vi "Calculate Thrust.vi"(8 "error in (no error)":errorcluster, 10 "Vessel in":refnum<class "Vessel.lvclass">, 11 "Thrust Allocation in":refnum<class "Thrust Allocation.lvclass">) -> (0 "error out":errorcluster, 2 "Vessel out":refnum<class "Vessel.lvclass">, 3 "Thrust Allocation out":refnum<class "Thrust Allocation.lvclass">)   [LabVIEW 2014, in "Thrust Allocation.lvclass"]
uses:
  Thrust Allocation.lvclass
  ROV/Vessel.lvclass
  <vilib>/Analysis/Matrix/Datatypes/RealMatrix.ctl
  <vilib>/Analysis/_algsub.llb/Real PseudoInverse Matrix.vi
  <vilib>/Analysis/baseanly.llb/A x Vector.vi
  <vilib>/Analysis/Matrix/Numeric/Multiply/Multiply - RM,R.vi
  <vilib>/Analysis/Matrix/Numeric/Conversions/Matrix To Array - RM.vi
  <vilib>/imath/engines/lvmath2/RunTimeEngine/IndexRead/NIMS M($,S).vi
  <instcachedir>/0/NIMS M($,S)_3E5749BBB62E49528D4765A77F1F6D98.lvgen/NIMS M($,S)_3E5749BBB62E49528D4765A77F1F6D98_000.vi
  <vilib>/imathl/engines/lvmath/Functions/Error Handling/Create Error.vi
  <vilib>/imath/engines/lvmath2/RunTimeEngine/BuiltInFunctions/length/NIMS_length(GV).vi
  <instcachedir>/0/NIMS_length(GV)_08A3D13377FD4E4B96F5795FBF3698FA.lvgen/NIMS_length(GV)_08A3D13377FD4E4B96F5795FBF3698FA_000.vi
  <vilib>/imath/engines/lvmath2/RunTimeEngine/RangeToken/NIMS_Range_R2 - Integer.vi
  <instcachedir>/0/NIMS_Range_R2 - Integer_2D1304BAF97744E0A293025746CBADFC.lvgen/NIMS_Range_R2 - Integer_2D1304BAF97744E0A293025746CBADFC_000.vi
  <vilib>/imath/engines/lvmath2/RunTimeEngine/CommandStatement/MC_CommandStatement_break.vi
  <vilib>/imath/engines/lvmath2/RunTimeEngine/IndexRead/NIMS V(S).vi
  <instcachedir>/0/NIMS V(S)_0488751826AF41519A22953C041130DC.lvgen/NIMS V(S)_0488751826AF41519A22953C041130DC_000.vi
  <vilib>/imath/engines/lvmath2/RunTimeEngine/VariableToken/NIMS_VariableToken_CondDefinedDefinedByReplace.vi
  <instcachedir>/0/NIMS_VariableToken_CondDefinedDefinedByReplace_D162CFFC24174562A9FEA619A91E1A56.lvgen/NIMS_VariableToken_CondDefinedDefinedByReplace_D162CFFC24174562A9FEA619A91E1A56_002.vi
  <vilib>/imath/engines/lvmath2/RunTimeEngine/IndexReplace/NIMS V(S)=S.vi
  <instcachedir>/0/NIMS V(S)=S_2D52C4EC15D8415E870AEE69FB516CCA.lvgen/NIMS V(S)=S_2D52C4EC15D8415E870AEE69FB516CCA_000.vi
  <vilib>/imath/engines/lvmath2/RunTimeEngine/ErrorHandling/NIMS_Create Error From Enums.vi
  <vilib>/imath/engines/lvmath2/RunTimeEngine/VariableToken/NIMS_VariableToken_CondDefined.vi
  <instcachedir>/0/NIMS_VariableToken_CondDefined_EE8DD211A89249938CE6537267F5C9B3.lvgen/NIMS_VariableToken_CondDefined_EE8DD211A89249938CE6537267F5C9B3_005.vi
  <vilib>/imath/engines/lvmath2/RunTimeEngine/NodeEndStatement/NIMS_NodeEndStatement_Output.vi
  <instcachedir>/0/NIMS_NodeEndStatement_Output_53EC0D466D134D7ABD903AC30B43404B.lvgen/NIMS_NodeEndStatement_Output_53EC0D466D134D7ABD903AC30B43404B_005.vi
  <vilib>/imath/engines/lvmath2/RunTimeEngine/ErrorHandling/NIMS_Finalize Error.vi
  Supervisor/Supervisor.lvclass
  Thruster/Thruster.lvclass
  <vilib>/Analysis/NI_AALPro.lvlib
  <vilib>/Analysis/NI_AALBase.lvlib
  <vilib>/Analysis/Matrix/NI_Matrix.lvlib
panel:
  in  "Numeric":dbl=1.0
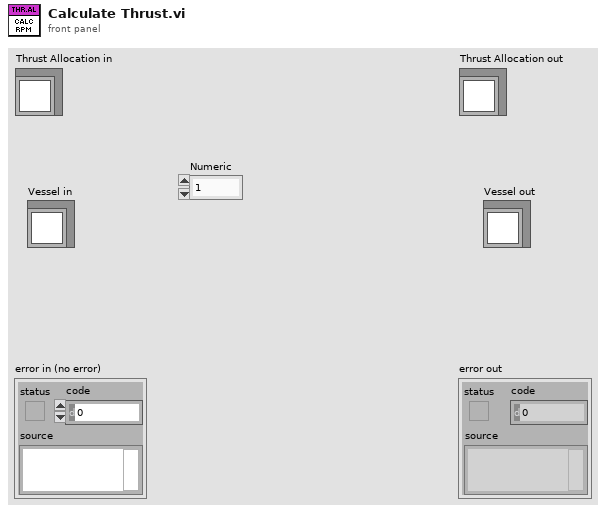
[diagram p1: front panel]
types:
  T1 = typedef "NI_Matrix.lvlib/RealMatrix.ctl" = dbl[][]
  T2 = cluster{"Measured":cluster{"Eta":dbl[], "Nu":dbl[], "Eta Dot":dbl[], "Nu Dot":dbl[]}, "Estimated":cluster{"Eta":dbl[], "Nu":dbl[], "Eta Dot":dbl[], "Nu Dot":dbl[]}, "Desired":cluster{"Eta":dbl[], "Nu":dbl[], "Eta Dot":dbl[], "Nu Dot":dbl[]}, "Previous Desired":cluster{"Eta":dbl[], "Nu":dbl[], "Eta Dot":dbl[], "Nu Dot":dbl[]}, "tau":dbl[], "Altitude":cluster{"Measured":dbl, "Estimated":dbl, "Desired":dbl, "Previous Desired":dbl, "Approximated":dbl, "grad F":dbl[]}, "rpm":dbl[], "Attitude":cluster{"Theta Measured":dbl[], "Theta Estimated":dbl[], "Omega Measured":dbl[], "Omega Estimated":dbl[], "Gyro Bias":dbl[]}}
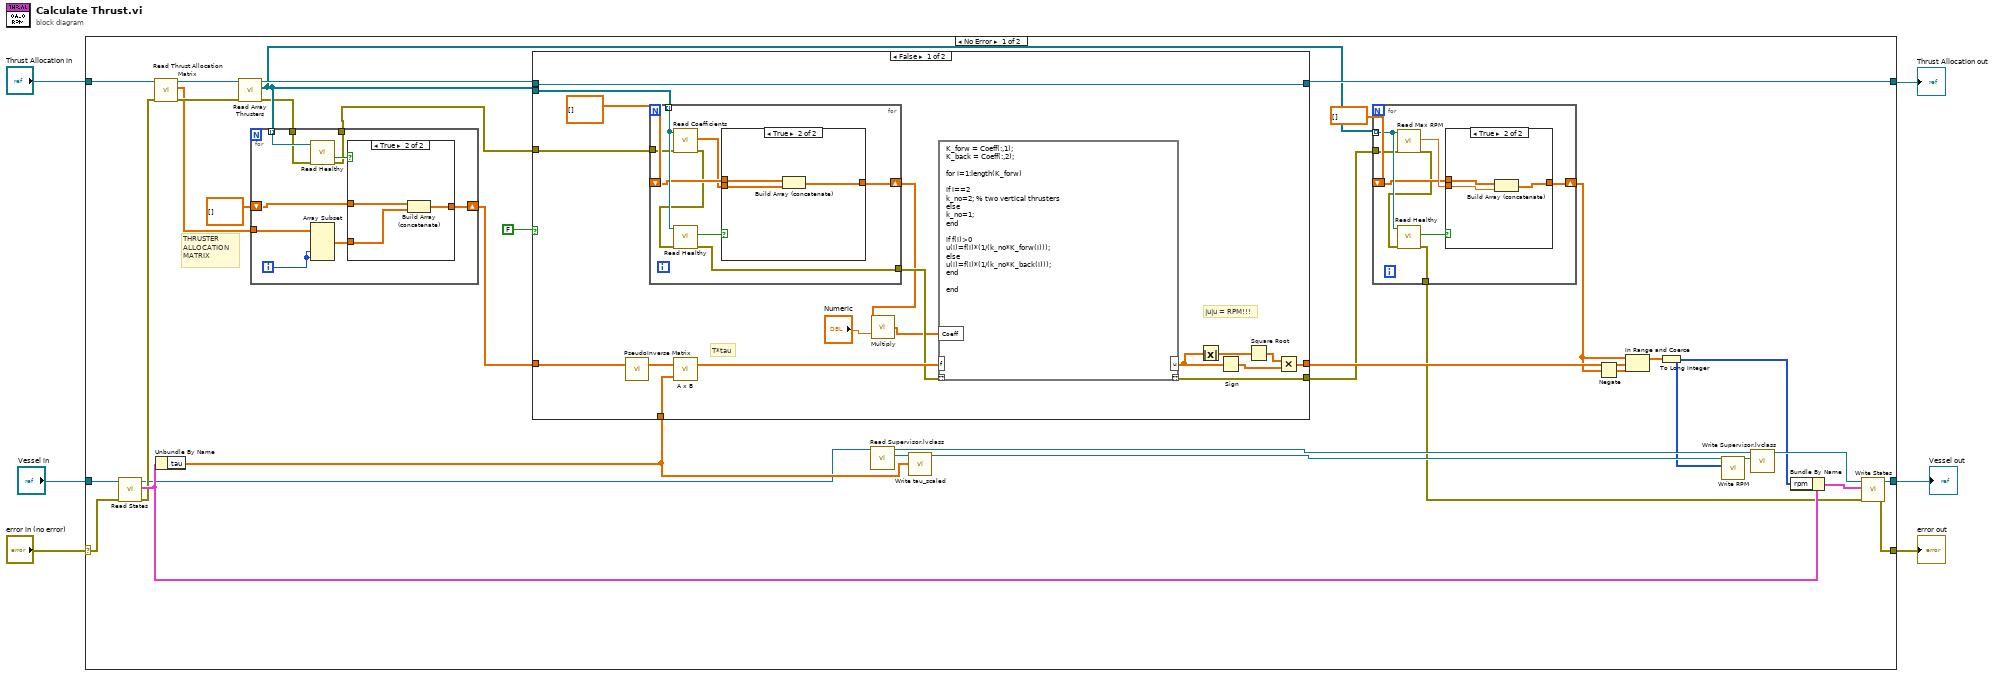
[diagram p0: block diagram]
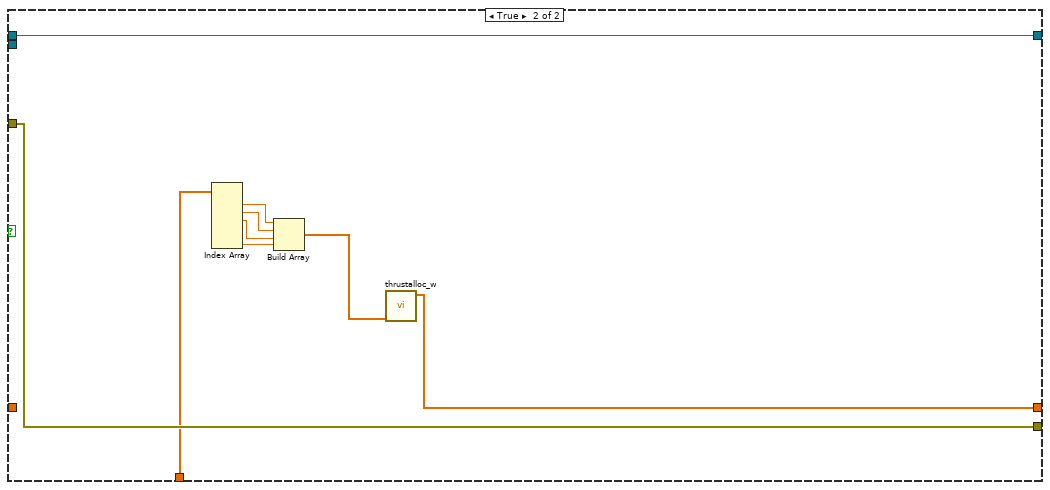
[diagram p3: hidden frame]
diagram:
  n1 = case shown="No Error" "error in (no error)" {
    selector: "error in (no error)" -> [w34 w345]
    tunnel: [w32 w345] -> w5
    tunnel: [w22 w344] -> w3
    tunnel: "Thrust Allocation in" -> [w25 w344]
    tunnel: "Vessel in" -> [w38 w343]
    tunnel: [w35 w343] -> w1
    frame No Error {
      # "THRUSTER\nALLOCATION\nMATRIX"
      n2 = call-dynamic "Read States.vi"("error in (no error)"=w34, "Vessel in"=w38) -> ("error out"=w24:errorcluster, "States"=w37:T2, "Vessel out"=w7:refnum<class "Vessel.lvclass">)  [unwired: 7 in]
      n3 = call-dynamic "Read Thrust Allocation Matrix.vi"("error in (no error)"=w24, "Thrust Allocation in"=w25) -> ("error out"=w33:errorcluster, "T"=w20:T1, "Thrust Allocation out"=w40:refnum<class "Thrust Allocation.lvclass">)  [unwired: 7 in]
      n4 = Unbundle By Name(w37) -> ("tau"=w8:dbl[])
      n5 = call "Read Array Thrusters.vi"("error in (no error)"=w33, "Thrust Allocation in"=w40) -> ("error out"=w16:errorcluster, "Array Thrusters"=w18:refnum<class "Thruster.lvclass">[], "Thrust Allocation out"=w23:refnum<class "Thrust Allocation.lvclass">)  [unwired: 7 in]
      n6 = for {
        shift-right: [w323] -> w19
        shift-left: T1 [] ("T") -> [w322]
        tunnel: w20 -> [w321]
        tunnel: w18 -> [w320] mode=indexing
        tunnel: w16 -> [w319]
        tunnel: [w318] -> w15
        i -> [w326]
        n7 = call-dynamic "Read Healthy.vi"("error in (no error)"=w319, "Thruster in"=w320) -> ("error out"=w318:errorcluster, "Healthy"=w324:bool)  [unwired: 7 in, 1 out]
        n8 = Array Subset(array=w321, index (col)=w326, length (col)=w326) -> (w325:T1)  [unwired: 2 in]
        n9 = case shown="True" w324 {
          tunnel: w325 -> [_ w330]
          tunnel: [w327 w329] -> w323
          tunnel: w322 -> [w327 w328]
          frame False {
          }
          frame True {
            n10 = Build Array (concatenate)(w328, w330) -> (w329:T1)
          }
        }
      }
      n11 = case shown="False" FALSE {
        tunnel: w8 -> [w58 w314]
        tunnel: w23 -> [w50 w317]
        tunnel: [w50 w317] -> w22
        tunnel: [w44 w315] -> w21
        tunnel: w19 -> [w55 _]
        tunnel: w18 -> [w54 _]
        tunnel: w15 -> [w53 w316]
        tunnel: [w52 w316] -> w13
        frame False {
          # "T*tau"
          # "|u|u = RPM!!!"
          n12 = call-poly <vilib>:"PseudoInverse Matrix.vi"("Input Matrix"=w55) -> ("PseudoInverse Matrix"=w57:T1)  [unwired: 1 in, 1 out]
          n13 = for {
            tunnel: w54 -> [w304] mode=indexing
            shift-right: [w302] -> w41
            shift-left: T1 [] ("Real Matrix") -> [w301]
            tunnel: w53 -> [w300]
            tunnel: [w298] -> w49
            n14 = call-dynamic "Read Coefficients.vi"("error in (no error)"=w300, "Thruster in"=w304) -> ("error out"=w299:errorcluster, "Coefficients"=w297:dbl[])  [unwired: 7 in, 1 out]
            n15 = call-dynamic "Read Healthy.vi"("error in (no error)"=w299, "Thruster in"=w304) -> ("error out"=w298:errorcluster, "Healthy"=w303:bool)  [unwired: 7 in, 1 out]
            n16 = case shown="True" w303 {
              tunnel: w297 -> [_ w308]
              tunnel: [w305 w307] -> w302
              tunnel: w301 -> [w305 w306]
              frame False {
              }
              frame True {
                n17 = Build Array (concatenate)(w306, w308) -> (w307:T1)
              }
            }
          }
          n18 = call-poly <vilib>:"A x B.vi"("Vector"=w58, "A"=w57) -> ("A x Vector"=w56:dbl[])  [unwired: 1 out]
          n19 = call-poly <vilib>:"Multiply.vi"("Real Scalar c"="Numeric", "Real Matrix A"=w41) -> ("A * c"=w42:T1)
          n20 = mathscript code="K_forw = Coeff(:,1);\nK_back = Coeff(:,2);\n\nfor i=1:length(K_forw)\n\nif i==2\nk_no=2; % two vertical thrusters\nelse\nk_no=1;\nend\n\nif f(i)>0\nu(i)=f(i)*(1/(k_no*K_forw(i)));\nelse\nu(i)=f(i)*(1/(k_no*K_back(i)));\nend\n\nend"("??"=w49, "Coeff"=w42, "f"=w56) -> ("??"=w52:errorcluster, "u"=w47:dbl[])
          n21 = Absolute Value(x=w47) -> (abs(x)=w48:dbl[])
          n22 = Sign(1:w47) -> (0:w45:dbl[])
          n23 = Square Root(x=w48) -> (sqrt(x)=w46:dbl[])
          n24 = Multiply(x=w46, y=w45) -> (x*y=w44:dbl[])
        }
        frame True {
          n25 = Index Array(array=w314) -> (element #1=w313:dbl, element #2=w312:dbl, element #3=w311:dbl, element #6=w310:dbl)  [unwired: 6 in, 2 out]
          n26 = Build Array(w313, w312, w311, w310) -> (w309:dbl[])
          n27 = call "thrustalloc_w.vi"("Forces and moments [N]/[Nm]"=w309) -> ("n [rpm]"=w315:dbl[])  [unwired: 10 in]
        }
      }
      n28 = call "Read Supervisor.lvclass.vi"("Vessel in"=w7) -> ("Supervisor.lvclass"=w29:refnum<class "Supervisor.lvclass">, "Vessel out"=w31:refnum<class "Vessel.lvclass">)  [unwired: 8 in, 1 out]
      n29 = call-dynamic "Write tau_scaled.vi"("tau_scaled"=w8, "Supervisor in"=w29) -> ("Supervisor out"=w28:refnum<class "Supervisor.lvclass">)  [unwired: 8 in, 1 out]
      n30 = for {
        tunnel: w18 -> [w337] mode=indexing
        shift-right: [w335] -> w17
        shift-left: dbl[] [] -> [w334]
        tunnel: w13 -> [w333]
        tunnel: [w331] -> w14
        n31 = call-dynamic "Read Max RPM.vi"("error in (no error)"=w333, "Thruster in"=w337) -> ("error out"=w332:errorcluster, "Max RPM"=w336:dbl)  [unwired: 7 in, 1 out]
        n32 = call-dynamic "Read Healthy.vi"("error in (no error)"=w332, "Thruster in"=w337) -> ("error out"=w331:errorcluster, "Healthy"=w338:bool)  [unwired: 7 in, 1 out]
        n33 = case shown="True" w338 {
          tunnel: w336 -> [_ w342]
          tunnel: [w339 w341] -> w335
          tunnel: w334 -> [w339 w340]
          frame False {
          }
          frame True {
            n34 = Build Array (concatenate)(w340, w342) -> (w341:dbl[])
          }
        }
      }
      n35 = Negate(x=w17) -> (-x=w39:dbl[])
      n36 = In Range and Coerce(upper limit=w17, x=w21, lower limit=w39) -> (coerced(x)=w9:dbl[])  [unwired: 1 out]
      n37 = To Long Integer(number=w9) -> (32bit integer=w26:i32[])
      n38 = call-dynamic "Write RPM.vi"("RPM"=w26, "Supervisor in"=w28) -> ("Supervisor out"=w27:refnum<class "Supervisor.lvclass">)  [unwired: 8 in, 1 out]
      n39 = call "Write Supervisor.lvclass.vi"("Supervisor.lvclass"=w27, "Vessel in"=w31) -> ("Vessel out"=w30:refnum<class "Vessel.lvclass">)  [unwired: 8 in, 1 out]
      n40 = Bundle By Name(cluster=w37, "rpm"=w26) -> (w36:T2)
      n41 = call-dynamic "Write States.vi"("error in (no error)"=w14, "States"=w36, "Vessel in"=w30) -> ("error out"=w32:errorcluster, "Vessel out"=w35:refnum<class "Vessel.lvclass">)  [unwired: 7 in]
    }
    frame Error {
    }
  }
  "error out" <- w5
  "Thrust Allocation out" <- w3
  "Vessel out" <- w1
